vi "parse and execute command.vi"(1 "Python Command":string="d:\\test.vi(gogo)") -> (0 "Python Return String":string="gogo")   [LabVIEW 2011]
panel:
  out "error out":errorcluster
  in  "VI Refnum":refnum<vi>
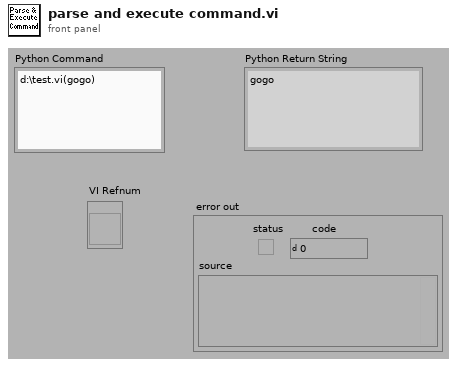
[diagram p1: front panel]
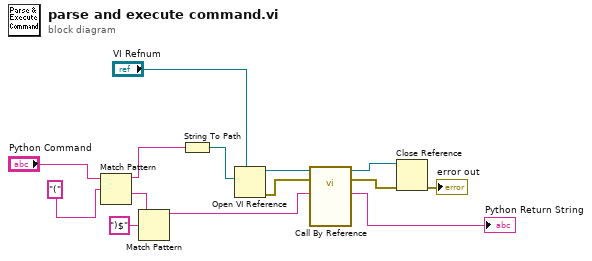
[diagram p0: block diagram]
diagram:
  n1 = Match Pattern(string="Python Command", regular expression="(") -> (before substring=w1:string, after substring=w11:string)  [unwired: 1 in, 2 out]
  n2 = Match Pattern(string=w11, regular expression=")$") -> (before substring=w5:string)  [unwired: 1 in, 3 out]
  n3 = String To Path(string=w1) -> (path=w2:path)
  n4 = Open VI Reference(type specifier VI Refnum (for type only)="VI Refnum", vi path=w2) -> (vi reference=w10:refnum<vi>, error out=w8:errorcluster)  [unwired: 4 in]
  n5 = call-by-ref "?"(reference=w10, error in=w8, "Input"=w5) -> (reference out=w9:refnum<vi>, error out=w7:errorcluster, "Output"=→"Python Return String":string)  [unwired: 9 in, 1 out]
  n6 = Close Reference(reference=w9, error in (no error)=w7) -> (error out=→"error out":errorcluster)
